vi "Coord window-Move to XYZ.vi"(8 "error in (no error)":errorcluster) -> (0 "error out":errorcluster)   [LabVIEW 2020]
uses:
  Globals/Coord window-Globals.vi
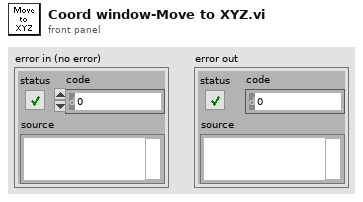
[diagram p1: front panel]
types:
  T1 = typedef "Coordinate list window refs.ctl" = cluster{"Window Name (i.e. Key)":string, "menu reference":refnum<k9>, "VI's reference":refnum<vi>, "Pane 1":refnum<vi>, "Pane 2":refnum<vi>, "Coord Listbox":refnum<vi>, "File name":refnum<vi>, "Picture Map":refnum<vi>, "Stage XYZ Position ind.":refnum<vi>}
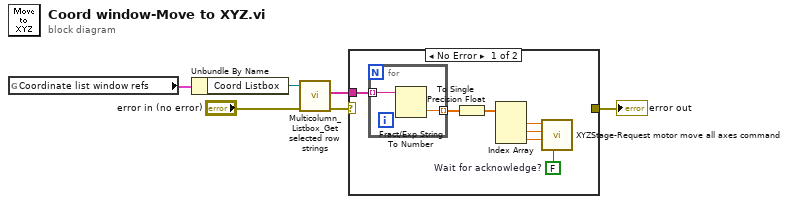
[diagram p0: block diagram]
diagram:
  n1 = global read "Coord window-Globals.vi" "Coordinate list window refs"() -> (w3:T1)
  n2 = Unbundle By Name(w3) -> ("Coord Listbox"=w2:refnum<vi>)
  n3 = call <userlib>:"Multicolumn_Listbox_Get selected row strings.vi"("error in (no error)"="error in (no error)", "MulticolumnListbox in"=w2) -> ("error out"=w5:errorcluster, "Selected row strings"=w4:string[])  [unwired: 7 in, 1 out]
  n4 = case shown="No Error" w5 {
    selector: w5 -> [_ w16]
    tunnel: w4 -> [w13 _]
    tunnel: [_ w16] -> w6
    frame No Error {
      w7 = FALSE  # Wait for acknowledge?
      n5 = for {
        tunnel: w13 -> [w15] mode=indexing
        tunnel: [w14] -> w12 mode=indexing
        n6 = Fract/Exp String To Number(string=w15) -> (number=w14:dbl)  [unwired: 3 in, 1 out]
      }
      n7 = To Single Precision Float(number=w12) -> (single precision float=w10:sgl[])
      n8 = Index Array(array=w10) -> (element #1=w11:sgl, element #2=w9:sgl, element #3=w8:sgl)  [unwired: 3 in]
      n9 = call "XYZStage-Request motor move all axes command.vi"("Wait for acknowledge?"=w7, "Motor Z"=w8, "Motor Y"=w9, "Motor X"=w11) -> ()  [unwired: 6 in, 2 out]
    }
    frame Error {
    }
  }
  "error out" <- w6
